vi "Configure Module.vi"(8 "error in":errorcluster, 10 "IOV ref in":variant, 11 "9210 in":refnum<class "9210.lvclass">) -> (0 "error out":errorcluster, 2 "IOV ref out":variant, 3 "9210 out":refnum<class "9210.lvclass">)   [LabVIEW 2020, in "Modules.lvlib" / "9210.lvclass"]
uses:
  9210.lvclass
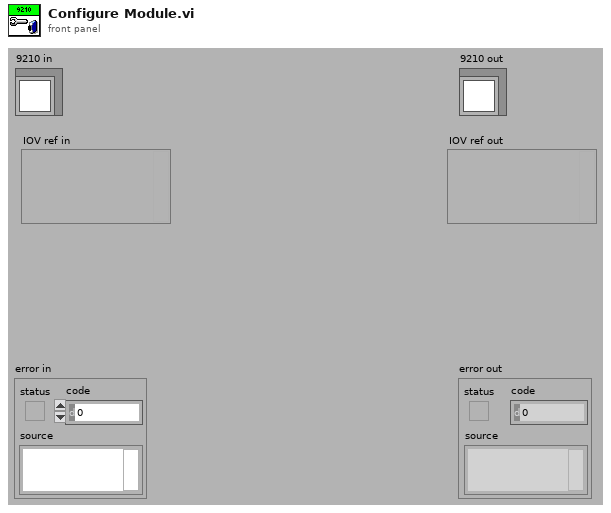
[diagram p1: front panel]
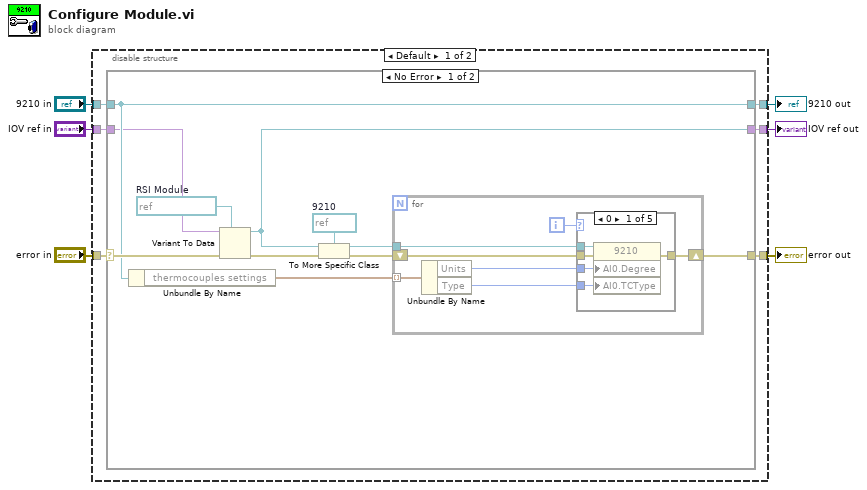
[diagram p0: block diagram]
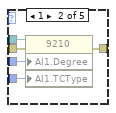
[diagram p2: hidden frame]
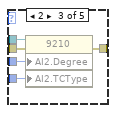
[diagram p3: hidden frame]
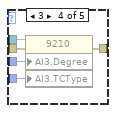
[diagram p4: hidden frame]
diagram:
  n1 = disable-structure shown="Default" {
    disable-tunnel: "error in" -> [w12 w57]
    disable-tunnel: [w11 w57] -> w5
    disable-tunnel: "9210 in" -> [w10 w55]
    disable-tunnel: [w9 w55] -> w3
    disable-tunnel: "IOV ref in" -> [w8 w56]
    disable-tunnel: [w7 w56] -> w1
    frame condition #0 {
      n2 = case shown="No Error" w12 {
        selector: w12 -> [w22 w54]
        tunnel: [w23 w54] -> w11
        tunnel: [w21 w53] -> w9
        tunnel: w10 -> [w21 w53]
        tunnel: w8 -> [w18 w52]
        tunnel: [w17 w52] -> w7
        frame No Error {
          w15 = refnum<k21> refnum  # 9210
          w16 = refnum<k21> refnum  # RSI Module
          n3 = Unbundle By Name(w21) -> ("thermocouples settings"=w20:cluster{"Units":u8, "Type":u8}[])
          n4 = Variant To Data(error in=w22, type=w16, Variant=w18) -> (data=w17:refnum<k21>, error out=w19:errorcluster)
          n5 = To More Specific Class(target class=w15, reference=w17, error in=w19) -> (specific class reference=w14:refnum<k21>, error out=w13:errorcluster)
          n6 = for {
            tunnel: w14 -> [w29]
            shift-right: [w30] -> w23
            shift-left: w13 -> [w28]
            tunnel: w20 -> [w26] mode=indexing
            i -> [w27]
            n7 = Unbundle By Name(w26) -> ("Units"=w25:u8, "Type"=w24:u8)
            n8 = case shown="0" w27 {
              tunnel: [w35 w40 w45 w50 w51] -> w30
              tunnel: w29 -> [w34 w39 w44 w49 _]
              tunnel: w28 -> [w33 w38 w43 w48 w51]
              tunnel: w24 -> [w32 w37 w42 w46 _]
              tunnel: w25 -> [w31 w36 w41 w47 _]
              frame 0 {
                n9 = property class="9210"(reference=w34, error in=w33, "AI0.Degree"=w31, "AI0.TCType"=w32) -> (error out=w35:errorcluster)  [unwired: 1 out]
              }
              frame 1 {
                n10 = property class="9210"(reference=w39, error in=w38, "AI1.Degree"=w36, "AI1.TCType"=w37) -> (error out=w40:errorcluster)  [unwired: 1 out]
              }
              frame 2 {
                n11 = property class="9210"(reference=w44, error in=w43, "AI2.Degree"=w41, "AI2.TCType"=w42) -> (error out=w45:errorcluster)  [unwired: 1 out]
              }
              frame 3 {
                n12 = property class="9210"(reference=w49, error in=w48, "AI3.Degree"=w47, "AI3.TCType"=w46) -> (error out=w50:errorcluster)  [unwired: 1 out]
              }
              frame Default {
              }
            }
          }
        }
        frame Error {
        }
      }
    }
    frame condition #1 (active) {
    }
  }
  "error out" <- w5
  "9210 out" <- w3
  "IOV ref out" <- w1
